vi "EventHandler-Change Order By Enter Key.vi"(5 "Next Ctrl":refnum<vi>, 7 "Controls for changing order":refnum<vi>[](array[refnum]), 9 "VKey":T1, 11 "Event Control":refnum<vi>) -> (3 "Discard?":bool)   [LabVIEW 2017]
doc: "Event handler that moves the input focus to the next control in Controls for changing order when the Enter key is pressed. Wire it into an event structure; Discard? reports whether the event should be discarded."
uses:
  <vilib>/event_ctls.llb/eventvkey.ctl
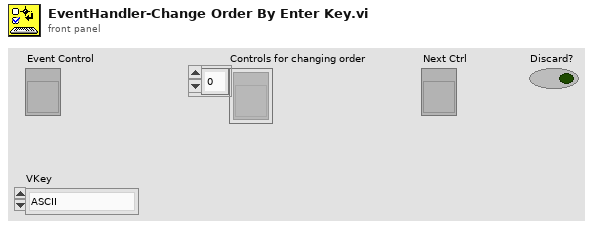
[diagram p1: front panel]
types:
  T1 = typedef "eventvkey.ctl" = enum16{"ASCII", "Enter", "Return", "Shift", "Ctrl", "Alt", "Cmd", "Opt", "Caps", "NumLock", "Clear", "Break", "Up", "Down", "Left", "Right", "Insert", "Delete", "Home", "End", "PageUp", "PageDown", "Escape", "Help", "Pause", "ScrollLock", "F1", "F2", "F3", "F4", "F5", "F6", "F7", "F8", "F9", "F10", "F11", "F12", "F13", "F14", "F15", "F16", "F17", "F18", "F19", "F20", "F21", "F22", "F23", "F24", "Play", "VolumeUp", "VolumeDown", "Mute", "Two Byte Char"}
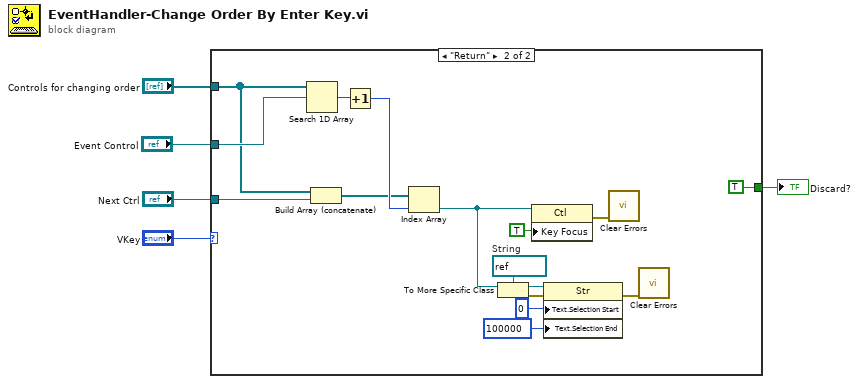
[diagram p0: block diagram]
diagram:
  n1 = case shown="\"Return\"" "VKey" {
    tunnel: [_ TRUE] -> w2
    tunnel: "Event Control" -> [_ w20]
    tunnel: "Controls for changing order" -> [_ w18]
    tunnel: "Next Ctrl" -> [_ w14]
    frame "ASCII", Default {
    }
    frame "Return" {
      w13 = refnum<vi> refnum  # String
      n2 = Search 1D Array(1D array=w18, element=w20) -> (index of element=w19:i32)  [unwired: 1 in]
      n3 = Build Array (concatenate)(w18, w14) -> (w15:refnum<vi>[])
      n4 = Increment(x=w19) -> (x+1=w17:i32)
      n5 = Index Array(array=w15, index=w17) -> (element=w9:refnum<vi>)
      n6 = To More Specific Class(target class=w13, reference=w9) -> (specific class reference=w12:refnum<vi>, error out=w8:errorcluster)  [unwired: 1 in]
      n7 = property class="Ctl"(reference=w9, "Key Focus"=TRUE) -> (error out=w7:errorcluster)  [unwired: 1 in, 1 out]
      n8 = property class="Str"(reference=w12, error in=w8, "Text.Selection Start"=u32 0 ("Text.Selection:Start"), "Text.Selection End"=u32 100000 ("Text.Selection:End")) -> (error out=w6:errorcluster)  [unwired: 1 out]
      n9 = call <vilib>:"Clear Errors.vi"("error in (no error)"=w7) -> ()  [unwired: 5 in, 2 out]
      n10 = call <vilib>:"Clear Errors.vi"("error in (no error)"=w6) -> ()  [unwired: 5 in, 2 out]
    }
  }
  "Discard?" <- w2
